vi "Adjust Dashboard Window.vi"(6 "Sizing Refnums":T1, 9 "Size Constraints":cluster{"min tab width":i32, "w/h":dbl}, 10 "VI":refnum<vi>, 11 "WIn Mode":refnum<notifier>) -> ()   [LabVIEW 2015]
uses:
  <vilib>/Utility/miscctls.llb/LVRectTypeDef.ctl
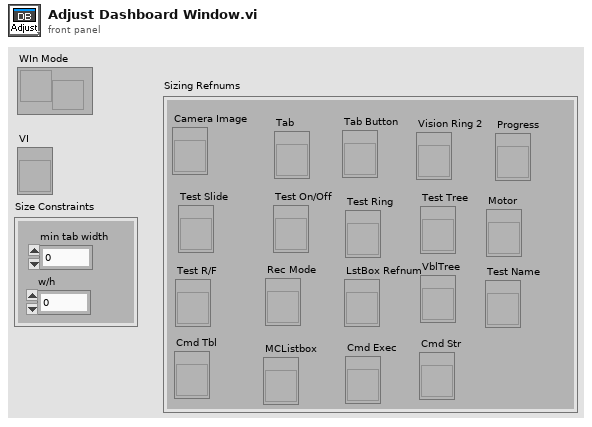
[diagram p1: front panel]
types:
  T1 = cluster{"Camera Image":refnum<vi>, "Tab":refnum<vi>, "Tab Button":refnum<vi>, "Vision Ring 2":refnum<vi>, "Rec Mode":refnum<vi>, "Test Slide":refnum<vi>, "Test On/Off":refnum<vi>, "Test Ring":refnum<vi>, "Test R/F":refnum<vi>, "Test Name":refnum<vi>, "Motor":refnum<vi>, "Progress":refnum<vi>, "LstBox Refnum":refnum<vi>, "Test Tree":refnum<vi>, "VblTree":refnum<vi>, "Cmd Tbl":refnum<vi>, "MCListbox":refnum<vi>, "Cmd Exec":refnum<vi>, "Cmd Str":refnum<vi>}
  T2 = typedef "LVRectTypeDef.ctl" = cluster{"Left":i16, "Top":i16, "Right":i16, "Bottom":i16}
  T3 = typedef "LVPointTypeDef.ctl" = cluster{"Horizontal":i16, "Vertical":i16}
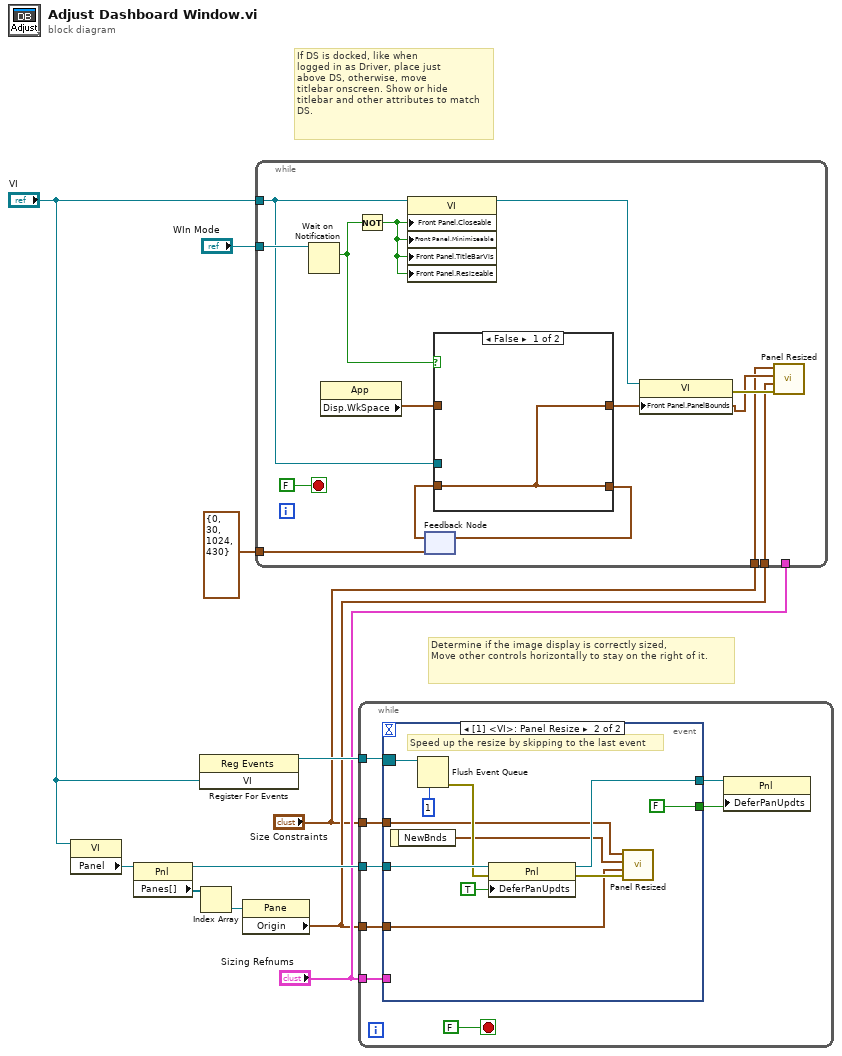
[diagram p0: block diagram]
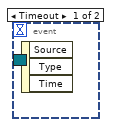
[diagram p2: hidden frame]
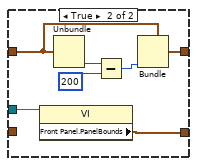
[diagram p3: hidden frame]
diagram:
  # "Determine if the image display is correctly sized,\nMove other controls horizontally to stay on the right of it."
  # "If DS is docked, like when\nlogged in as Driver, place just\nabove DS, otherwise, move\ntitlebar onscreen. Show or hide\ntitlebar and other attributes to match\nDS."
  n1 = property class="VI"(reference="VI") -> ("Panel"=w8:refnum<vi>)  [unwired: 1 in, 2 out]
  n2 = property class="Pnl"(reference=w8) -> (reference out=w5:refnum<vi>, "Panes[]"=w7:refnum<vi>[])  [unwired: 1 in, 1 out]
  n3 = register-events("VI") -> (reference out=w10:refnum<event-registration>)  [unwired: 2 in, 1 out]
  n4 = Index Array(array=w7) -> (element=w6:refnum<vi>)  [unwired: 1 in]
  n5 = property class="Pane"(reference=w6) -> ("Origin"=w3:T3)  [unwired: 1 in, 2 out]
  n6 = while {
    tunnel: "WIn Mode" -> [w24]
    tunnel: "VI" -> [w16]
    tunnel: "Sizing Refnums" -> [_]
    tunnel: w3 -> [w20]
    tunnel: "Size Constraints" -> [w18]
    tunnel: T2 {"Left"=0, "Top"=30, "Right"=1024, "Bottom"=430} ("Front Panel.PanelBounds") -> [w13]
    stop <- FALSE stop-if-true
    n7 = Wait on Notification(notifier=w24) -> (notification=w17:bool)  [unwired: 3 in, 3 out]
    n8 = property class="App"() -> ("Disp.WkSpace"=w23:T2)  [unwired: 2 in, 2 out]
    n9 = Not(x=w17) -> (.not. x?=w12:bool)
    n10 = property class="VI"(reference=w16, "Front Panel.Closeable"=w12, "Front Panel.Minimizeable"=w12, "Front Panel.TitleBarVis"=w12, "Front Panel.Resizeable"=w12) -> (reference out=w22:refnum<vi>)  [unwired: 1 in, 1 out]
    n11 = feedback #1(w13) -> (w14:T2)
    n12 = case shown="False" w17 {
      tunnel: w23 -> [_ w29]
      tunnel: [w26 w30] -> w19
      tunnel: w16 -> [_ w28]
      tunnel: [w26 w27] -> w15
      tunnel: w14 -> [w26 _]
      frame False {
      }
      frame True {
        n13 = property class="VI"(reference=w28) -> ("Front Panel.PanelBounds"=w27:T2)  [unwired: 1 in, 2 out]
        n14 = Unbundle(w29) -> ("Bottom"=w33:i16)  [unwired: 3 out]
        n15 = Subtract(x=w33, y=200) -> (x-y=w31:i32)
        n16 = Bundle(cluster=w29, "Bottom"=w31) -> (w30:T2)  [unwired: 3 out]
      }
    }
    n17 = feedback-in #1(w15) -> ()
    n18 = property class="VI"(reference=w22, "Front Panel.PanelBounds"=w19) -> (error out=w21:errorcluster)  [unwired: 1 in, 1 out]
    n19 = call "Panel Resized.vi"("error in (no error)"=w21, "Origin"=w20, "NewBnds"=w19, "Size Constraints"=w18) -> ()  [unwired: 7 in, 1 out]
  }
  n20 = while {
    tunnel: w10 -> [w40]
    tunnel: "Sizing Refnums" -> [w39]
    tunnel: "Size Constraints" -> [w38]
    tunnel: w3 -> [w37]
    tunnel: w5 -> [w36]
    stop <- FALSE stop-if-true
    n21 = event shown="[1] <VI>: Panel Resize" {
      selector: w40 -> [_ w49]
      dyn-events: _ -> [_ _]
      timeout: _ -> [_ _]
      tunnel: w39 -> [_ _]
      tunnel: w38 -> [_ w44]
      tunnel: w37 -> [_ w42]
      tunnel: w36 -> [_ w52]
      tunnel: [_ FALSE ("Defer Panel Updates")] -> w35
      tunnel: [_ w46] -> w34
      event Timeout {
        n22 = event-data() -> ()  [unwired: 1 in, 3 out]
      }
      event Panel Resize {
        # "Speed up the resize by skipping to the last event"
        n23 = event-data() -> ("NewBnds"=w43:T2)  [unwired: 1 in]
        n24 = Flush Event Queue(0:w49, 5:1 ("keep most recent")) -> (11:w47:errorcluster)  [unwired: 4 in, 2 out]
        n25 = property class="Pnl"(reference=w52, error in=w47, "DeferPanUpdts"=TRUE ("Defer Panel Updates")) -> (reference out=w46:refnum<vi>, error out=w45:errorcluster)
        n26 = call "Panel Resized.vi"("error in (no error)"=w45, "Origin"=w42, "NewBnds"=w43, "Size Constraints"=w44) -> ()  [unwired: 7 in, 1 out]
      }
    }
    n27 = property class="Pnl"(reference=w34, "DeferPanUpdts"=w35) -> ()  [unwired: 1 in, 2 out]
  }
